vi "sc_unix_time.vi"() -> (2 "seconds since 1Jan1904":timestamp, 3 "Numeric":dbl)   [LabVIEW 2018]
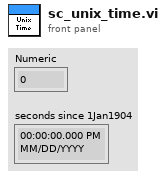
[diagram p1: front panel]
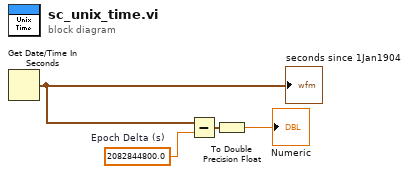
[diagram p0: block diagram]
diagram:
  w2 = 2082844800.0  # Epoch Delta (s)
  n1 = Get Date/Time In Seconds() -> (seconds since 1Jan1904=w4:timestamp)
  "seconds since 1Jan1904" <- w4
  n2 = Subtract(x=w4, y=w2) -> (x-y=w1:timestamp)
  n3 = To Double Precision Float(number=w1) -> (double precision float=→"Numeric":dbl)
